vi "RelativePos.vi"(11 "AxisPos":dbl[](array[numeric])) -> (3 "Relative Position":dbl[](array[numeric]))   [LabVIEW 2019]
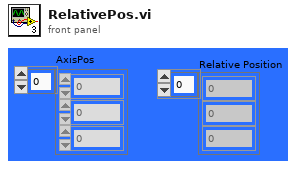
[diagram p1: front panel]
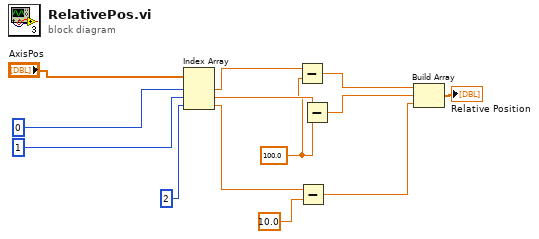
[diagram p0: block diagram]
diagram:
  w10 = 100.0 ("y")
  n1 = Index Array(array="AxisPos", index #1=0 ("index"), index #2=1 ("index"), index #3=2 ("index")) -> (element #1=w1:dbl, element #2=w11:dbl, element #3=w4:dbl)
  n2 = Subtract(x=w1, y=w10) -> (x-y=w9:dbl)
  n3 = Subtract(x=w4, y=10.0) -> (x-y=w2:dbl)
  n4 = Subtract(x=w11, y=w10) -> (x-y=w8:dbl)
  n5 = Build Array(w9, w8, w2) -> (→"Relative Position":dbl[])
